vi "Read FunctionCreateSocketHandler.vi"(8 "error in (no error)":errorcluster, 11 "Logger in":refnum<class "Logger.lvclass">) -> (0 "error out":errorcluster, 2 "FunctionCreateSocketHandler":string="create_socket_handler", 3 "Logger out":refnum<class "Logger.lvclass">)   [LabVIEW 2022 SP3, in "Logger.lvlib" / "Logger.lvclass"]
uses:
  Logger.lvclass
  Logger.lvclass/Logger.ctl
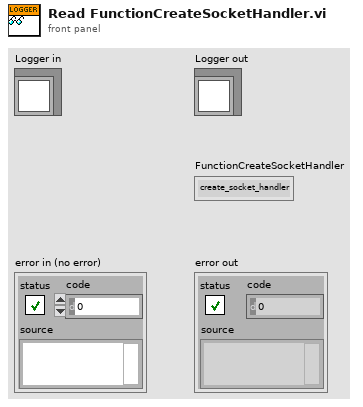
[diagram p1: front panel]
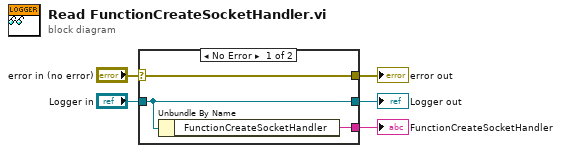
[diagram p0: block diagram]
diagram:
  n1 = case shown="No Error" "error in (no error)" {
    selector: "error in (no error)" -> [w8 w9]
    tunnel: [w8 w9] -> w4
    tunnel: [w7 w10] -> w2
    tunnel: "Logger in" -> [w7 w10]
    tunnel: [w6 _] -> w1
    frame No Error {
      n2 = Unbundle By Name(w7) -> ("FunctionCreateSocketHandler"=w6:string)
    }
    frame Error {
    }
  }
  "error out" <- w4
  "Logger out" <- w2
  "FunctionCreateSocketHandler" <- w1
